vi "daqio_Get_All_Device_Types.vi"(8 "error in (no error)":errorcluster, 11 "daq.io type in":T6={"daq.io ref"=refnum, "daq.io API Base"="http://dashboard.daq.io/api/v1", "Device Type Key"="", "Device Key"="", "Account ID"=""}) -> (0 "error out":errorcluster, 2 "Device Types":T1[](array[typedef]), 3 "daq.io type out":T6={"daq.io ref"=refnum, "daq.io API Base"="http://dashboard.daq.io/api/v1", "Device Type Key"="", "Device Key"="", "Account ID"=""})   [LabVIEW 2013, in "daqio minimal.lvlib"]
doc: "This VI returns all Device Types associated with the logged in user on this account.\nThis returns a potentially large JSON document over the network. When only limited bandwidth is available, try more specific fucntions such as \"Get Specific Device Type\" or similar."
uses:
  daqio minimal.lvlib
  _typedefs/daqio-Type.ctl
  <vilib>/httpClient/ClientHandle.ctl
  _typedefs/daqio-Device-Type-Info-return.ctl
  _typedefs/daqio-Channel-Type-POST-return.ctl
  _typedefs/daqio-Device.ctl
  _typedefs/daqio-Event-Type.ctl
  _typedefs/daqio-Tag-Type-POST-return.ctl
  <vilib>/Easy HTTP Client/Easy HTTP.lvlib
  <vilib>/httpClient/LabVIEWHTTPClient.lvlib
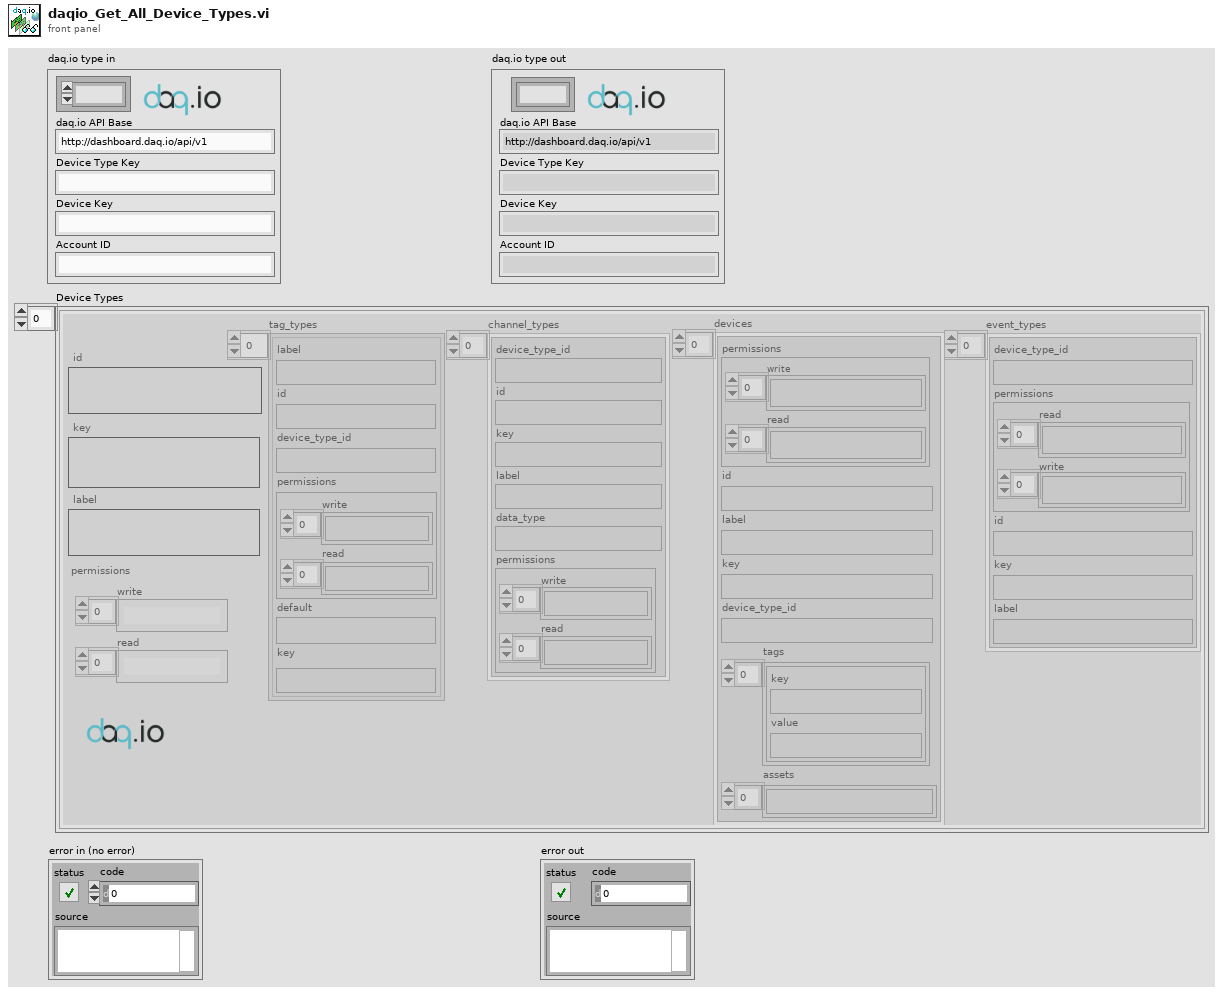
[diagram p1: front panel]
types:
  T1 = typedef "daqio minimal.lvlib/daqio-Device-Type-Info-return.ctl" = cluster{"channel_types":T2[], "devices":T3[], "label":string, "event_types":T4[], "key":string, "tag_types":T5[], "id":string, "permissions":cluster{"write":string[], "read":string[]}}
  T2 = typedef "daqio minimal.lvlib/daqio-Channel-Type-POST-return.ctl" = cluster{"device_type_id":string, "id":string, "key":string, "label":string, "data_type":string, "permissions":cluster{"write":string[], "read":string[]}}
  T3 = typedef "daqio minimal.lvlib/daqio-Device.ctl" = cluster{"permissions":cluster{"write":string[], "read":string[]}, "id":string, "label":string, "key":string, "device_type_id":string, "tags":cluster{"key":string, "value":string}[], "assets":string[]}
  T4 = typedef "daqio minimal.lvlib/daqio-Event-Type.ctl" = cluster{"device_type_id":string, "permissions":cluster{"read":string[], "write":string[]}, "id":string, "key":string, "label":string}
  T5 = typedef "daqio minimal.lvlib/daqio-Tag-Type-POST-return.ctl" = cluster{"label":string, "id":string, "device_type_id":string, "permissions":cluster{"write":string[], "read":string[]}, "default":string, "key":string}
  T6 = typedef "daqio minimal.lvlib/daqio-Type.ctl" = cluster{"daq.io ref":T7, "daq.io API Base":string, "Device Type Key":string, "Device Key":string, "Account ID":string}
  T7 = typedef "LabVIEWHTTPClient.lvlib/ClientHandle.ctl" = refnum<k1>
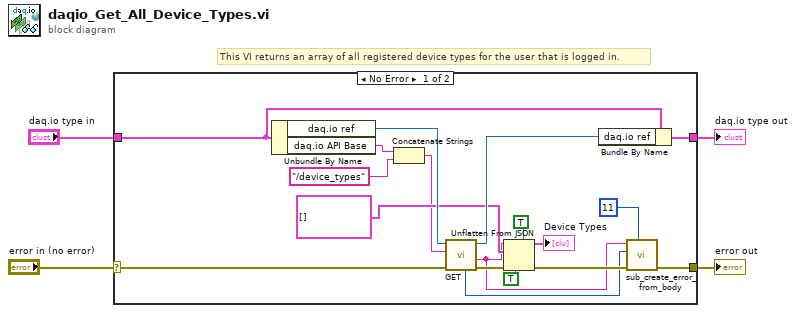
[diagram p0: block diagram]
diagram:
  # "This VI returns an array of all registered device types for the user that is logged in."
  n1 = case shown="No Error" "error in (no error)" {
    selector: "error in (no error)" -> [w18 w23]
    tunnel: "daq.io type in" -> [w22 w24]
    tunnel: [w21 w24] -> w3
    tunnel: [w8 w23] -> w2
    frame No Error {
      n2 = Unbundle By Name(w22) -> ("daq.io ref"=w20:T7, "daq.io API Base"=w16:string)
      n3 = Concatenate Strings(w16, "/device_types") -> (w13:string)
      n4 = call <vilib>:"GET.vi"("error in (no error)"=w18, "url"=w13, "client handle"=w20) -> ("error out"=w17:errorcluster, "body"=w5:string, "client handle out"=w19:T7, "HTTP Response Code"=w7:i32)  [unwired: 4 in, 1 out]
      n5 = Unflatten From JSON(enable LabVIEW extensions? (T)=TRUE, JSON string=w5, type and defaults=T1[] [], default null elements? (F)=TRUE, error in (no error)=w17) -> (value=→"Device Types":T1[], error out=w9:errorcluster)  [unwired: 2 in]
      n6 = Bundle By Name(cluster=w22, "daq.io ref"=w19) -> (w21:T6)
      n7 = call "sub_create_error_from_body.vi"("error code"=11, "error in (no error)"=w9, "http code"=w7, "body"=w5) -> ("error out"=w8:errorcluster)  [unwired: 7 in]
    }
    frame Error {
    }
  }
  "error out" <- w2
  "daq.io type out" <- w3
